vi "Check WavL Type(SubVI).vi"(0 "N systems":i32, 5 "Lambda, nm":i32[](array[numeric]), 11 "error in":errorcluster) -> (4 "all NonRed":bool, 6 "all Red":bool, 8 "all NewRed":bool, 10 "all OldRed":bool, 15 "error out":errorcluster)   [LabVIEW 2017]
panel:
  # "Inputs"
  # "Outputs"
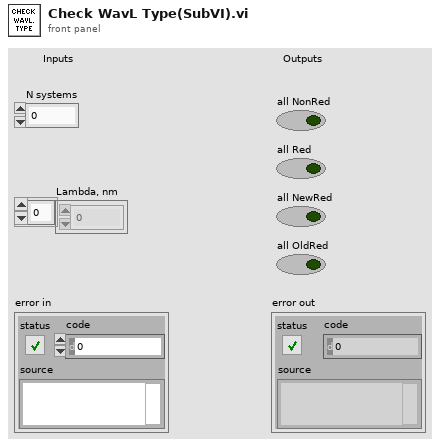
[diagram p1: front panel]
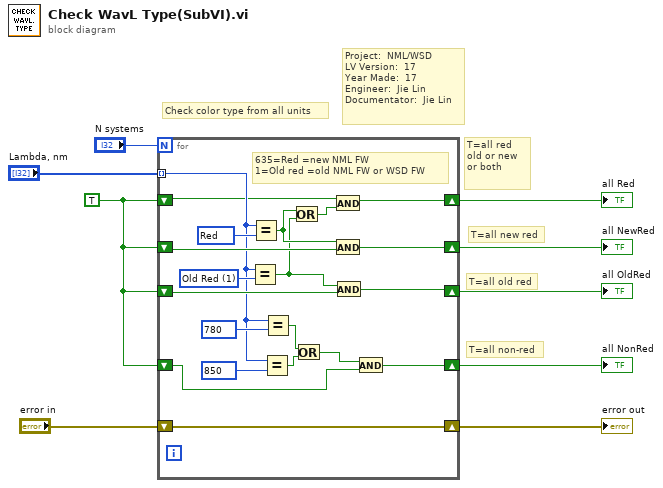
[diagram p0: block diagram]
diagram:
  w5 = TRUE
  # "Project:  NML/WSD \nLV Version:  17\nYear Made:  17\nEngineer:  Jie Lin\nDocumentator:  Jie Lin"
  # "T=all red \nold or new or both"
  # "T=all non-red"
  # "T=all old red"
  # "T=all new red"
  # "Check color type from all units"
  n1 = for {
    N: "N systems" -> [_]
    tunnel: "Lambda, nm" -> [w18] mode=indexing
    shift-right: [w28] -> w8
    shift-left: w5 -> [w27]
    shift-right: [w25] -> w9
    shift-left: w5 -> [w26]
    shift-right: [w17] -> w6
    shift-left: w5 -> [w16]
    shift-right: [w12] -> w7
    shift-left: w5 -> [w11]
    shift-right: [w10] -> w1
    shift-left: "error in" -> [w10]
    w22 = 850 items=["None"=0, "Red"=635, "780"=780, "850"=850, "Old Red"=1, "No Connect"=2]
    w23 = 780 items=["None"=0, "Red"=635, "780"=780, "850"=850, "Old Red"=1, "No Connect"=2]
    w24 = 1 items=["None"=0, "Red"=635, "780"=780, "850"=850, "Old Red"=1, "No Connect"=2]
    w29 = 635 items=["None"=0, "Red"=635, "780"=780, "850"=850, "Old Red"=1, "No Connect"=2]
    # "635=Red =new NML FW\n1=Old red =old NML FW or WSD FW"
    n2 = Equal?(x=w18, y=w24) -> (x = y?=w14:bool)
    n3 = Equal?(x=w18, y=w29) -> (x = y?=w15:bool)
    n4 = Equal?(x=w18, y=w22) -> (x = y?=w20:bool)
    n5 = Equal?(x=w18, y=w23) -> (x = y?=w21:bool)
    n6 = Or(x=w15, y=w14) -> (x .or. y?=w13:bool)
    n7 = Or(x=w21, y=w20) -> (x .or. y?=w19:bool)
    n8 = And(x=w11, y=w13) -> (x .and. y?=w12:bool)
    n9 = And(x=w15, y=w27) -> (x .and. y?=w28:bool)
    n10 = And(x=w14, y=w26) -> (x .and. y?=w25:bool)
    n11 = And(x=w19, y=w16) -> (x .and. y?=w17:bool)
  }
  "all OldRed" <- w9
  "all NewRed" <- w8
  "all Red" <- w7
  "all NonRed" <- w6
  "error out" <- w1
